vi "latest scan file.vi"(7 "source":enum16{"last scan file", "manual"}(ring)=enum."manual", 10 "file path in":path, 11 "sweep folder":path=path "E:/data/Ultrasound/Experiment/ProbeTest/Probe10/YBCO_5/sweep7") -> (0 "temperature (K)":dbl, 1 "file or folder exists?":bool, 2 "file path out":path, 3 "Magn Field (T)":dbl)   [LabVIEW 2015]
uses:
  ctl -- name dispatcher -- action.ctl
  file -- scan filename.ctl
  file -- scan filename action.ctl
  file -- 9w path.vi
  <vilib>/Utility/file.llb/Read From Spreadsheet File (string).vi
panel:
  in  "coerse with sweep folder?":bool=TRUE
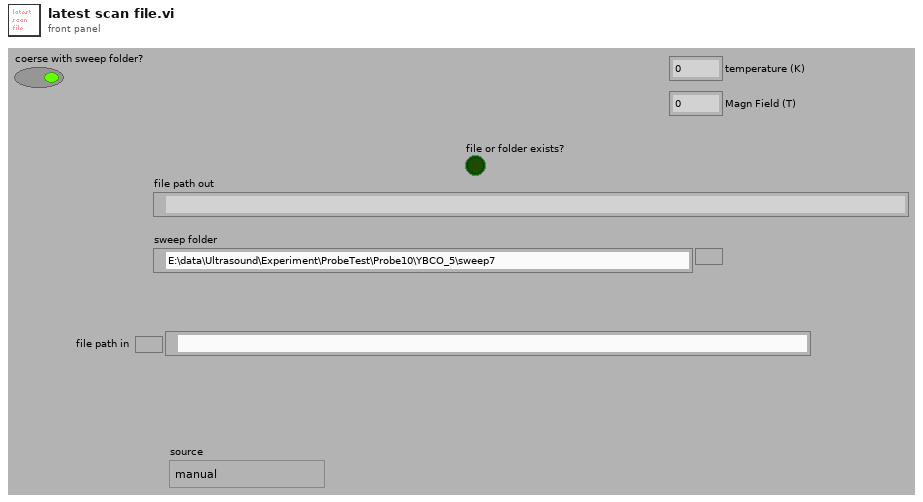
[diagram p1: front panel]
types:
  T1 = typedef "ctl -- name dispatcher -- action.ctl" = enum16{"peak frequency", "peak frequency DUMP", "peak gamma DUMP", "peak gamma", "peak frequency TEST", "peak gamma TEST", "ultrasonic power", "time in gamma", "set temperature ", "set temperature timer", "peak default gamma", "last scan file", "peak freq gamma TEST", "peak NAMES", "errors", "P_I_D", "P", "I", "D", "power vs time", "power vs time TIMER", "void", "power log", "set temperature - SINE", "itc ltc log", "peak - time in gamma"}
  T2 = typedef "file -- scan filename action.ctl" = enum16{"prefix base name", "datestring regexp", "parse datestring", "datestring", "filename regexp", "parse filename", "datestring regexp (no brackets)", "suffix base name"}
  T3 = typedef "file -- scan filename.ctl" = cluster{"mmddyy (str)":string, "counter (str)":string, "to F (kHz)":dbl, "from F (kHz)":dbl, "temperature (K)":dbl, "date/time string":string, "time stamp":timestamp, "base name":string, "temperature (str)":string, "from F (str)":string, "to F (str)":string, "format":enum16{"no date string", "with date string"}, "power (V)":dbl, "power (str) ":string, "Magn Field (T)":dbl, "Magn Field (str)":string}
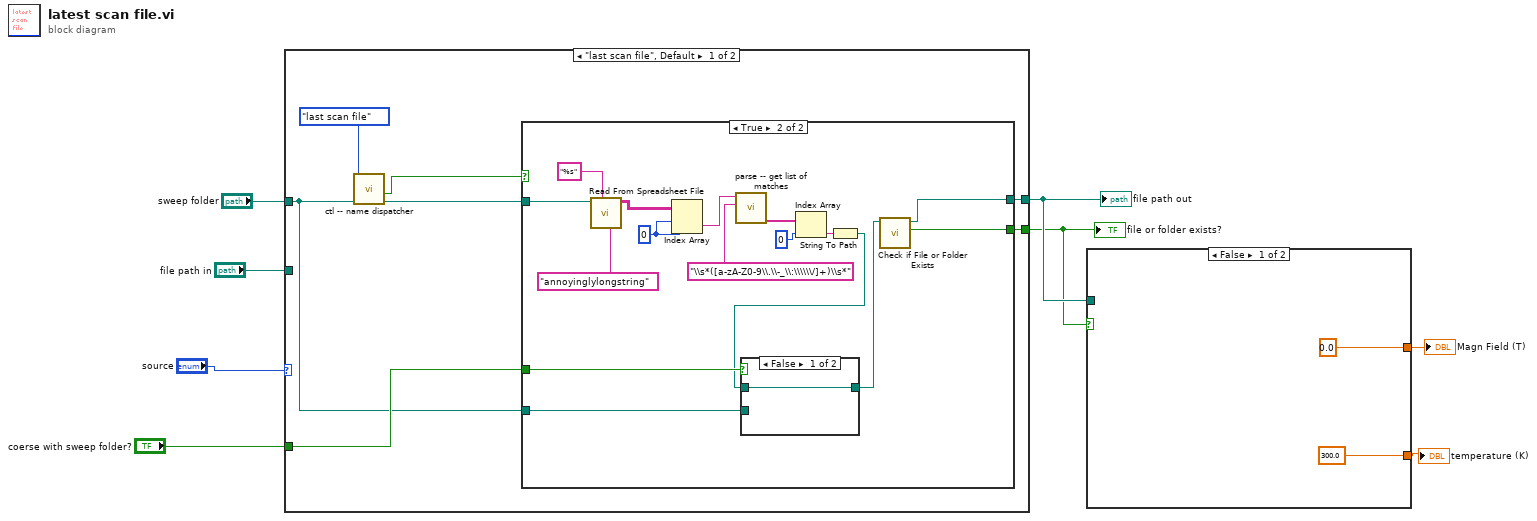
[diagram p0: block diagram]
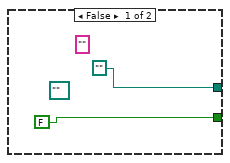
[diagram p2: hidden frame]
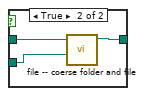
[diagram p3: hidden frame]
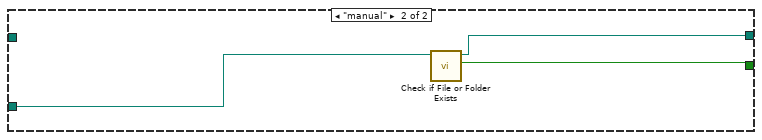
[diagram p4: hidden frame]
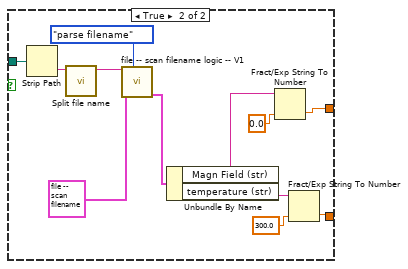
[diagram p5: hidden frame]
diagram:
  n1 = case shown="\"last scan file\", Default" "source" {
    tunnel: "sweep folder" -> [w12 _]
    tunnel: [w15 w39] -> w7
    tunnel: [w14 w38] -> w5
    tunnel: "file path in" -> [_ w40]
    tunnel: "coerse with sweep folder?" -> [w13 _]
    frame "last scan file", Default {
      n2 = call "ctl -- name dispatcher.vi"("sweep folder path"=w12, "ctl name dispatch"=ctl_--_name_dispatcher_--_action."last scan file" ("ctl kind")) -> ("file path"=w9:path, "file or folder exists?"=w10:bool)  [unwired: 7 in, 1 out]
      n3 = case shown="True" w10 {
        tunnel: w9 -> [_ w33]
        tunnel: [FALSE w24] -> w14
        tunnel: [path "" w23] -> w15
        tunnel: w12 -> [_ w21]
        tunnel: w13 -> [_ w20]
        frame False {
          (unwired) "" ("format (%s)")
          (unwired) path "" ("dup path")
        }
        frame True {
          w29 = 0 ("disabled index (col)")
          n4 = call-poly <vilib>:"Read From Spreadsheet File.vi"("delimiter (\\t)"="annoyinglylongstring" ("delimiter (\\t)"), "format (%s)"="%s", "file path (dialog if empty)"=w33) -> ("all rows"=w30:string[][])  [unwired: 4 in, 4 out]
          n5 = Index Array(array=w30, index (row)=w29, index (col)=w29) -> (element=w28:string)
          n6 = call "parse -- get list of matches.vi"("regexp"="\\s*([a-zA-Z0-9\\.\\-_\\:\\\\\\/]+)\\s*", "string"=w28) -> ("Array"=w26:string[])  [unwired: 7 in, 2 out]
          n7 = Index Array(array=w26, index=0) -> (element=w22:string)
          n8 = String To Path(string=w22) -> (path=w19:path)
          n9 = case shown="False" w20 {
            tunnel: w19 -> [w34 w37]
            tunnel: w21 -> [_ w36]
            tunnel: [w34 w35] -> w18
            frame False {
            }
            frame True {
              n10 = call "file -- coerse folder and file.vi"("sweep folder"=w36, "file"=w37) -> ("sweep file"=w35:path)  [unwired: 9 in]
            }
          }
          n11 = call <vilib>:"Check if File or Folder Exists.vi"("path"=w18) -> ("file or folder exists?"=w24:bool, "dup path"=w23:path)  [unwired: 8 in, 1 out]
        }
      }
    }
    frame "manual" {
      n12 = call <vilib>:"Check if File or Folder Exists.vi"("path"=w40) -> ("file or folder exists?"=w38:bool, "dup path"=w39:path)  [unwired: 8 in, 1 out]
    }
  }
  "file or folder exists?" <- w5
  "file path out" <- w7
  n13 = case shown="False" w5 {
    tunnel: w7 -> [_ w51]
    tunnel: [300.0 w50] -> w6
    tunnel: [0.0 w43] -> w1
    frame False {
    }
    frame True {
      n14 = Strip Path(path=w51) -> (name=w52:string)  [unwired: 1 out]
      n15 = call "Split file name.vi"("file name"=w52) -> ("name"=w49:string)  [unwired: 8 in, 2 out]
      n16 = call "file -- scan filename logic -- V1.vi"("scan fileneme action"=file_--_scan_filename_action."parse filename", "scan filename IN"=T3 {"mmddyy (str)"="", "counter (str)"="", "to F (kHz)"=0.0, "from F (kHz)"=0.0, "temperature (K)"=0.0, "date/time string"="", "time stamp"=timestamp(19856294.882018566 s since 1904-01-01), "base name"="", "temperature (str)"="", "from F (str)"="", "to F (str)"="", "format"=enum."no date string", "power (V)"=0.0, "power (str) "="", "Magn Field (T)"=0.0, "Magn Field (str)"=""}, "base name IN"=w49) -> ("scan filename OUT"=w47:T3)  [unwired: 6 in, 2 out]
      n17 = Unbundle By Name(w47) -> ("Magn Field (str)"=w44:string, "temperature (str)"=w53:string)
      n18 = Fract/Exp String To Number(string=w44, default (0 dbl)=0.0 ("default (0 DBL)")) -> (number=w43:dbl)  [unwired: 2 in, 1 out]
      n19 = Fract/Exp String To Number(string=w53, default (0 dbl)=300.0 ("default (0 DBL)")) -> (number=w50:dbl)  [unwired: 2 in, 1 out]
    }
  }
  "temperature (K)" <- w6
  "Magn Field (T)" <- w1
